vi "Modbus.vi"(8 "Command":string="\n", 10 "VISA资源名称":refnum<visa-resource-name>="COM1") -> (1 "响应":string)   [LabVIEW 2017]
uses:
  Program Files (x86)/National Instruments/LabVIEW 2017/examples/Instrument IO/Serial/support/Serial - Settings.ctl
  <vilib>/Instr/_visa.llb/VISA Configure Serial Port (Instr).vi
  <vilib>/NI/Modbus Library/API/Master/Modbus Master.lvclass
  <vilib>/NI/Modbus Library/API/Wrapper/Create Serial Master.vi
  <vilib>/NI/Modbus Library/API/Wrapper/API Main.lvlib
panel:
  out "字符串":string
  in  "register values 2":u16[](array[numeric])
  out "register values":u16[](array[numeric])
  out "error out":errorcluster
  in  "VISA resource name":refnum<visa-resource-name>
  out "Value 2":string
  out "Value":string
  out "子字符串":string
  in  "串口设置":T1={"波特率"=9600, "数据位"=8, "校验"=enum."None", "停止位"=10, "流控制"=0} {"流控制" items=["无"=0, "XON/XOFF"=1, "RTS/CTS"=2, "DTR/DSR"=4]; "停止位" items=["1.0"=10, "1.5"=15, "2.0"=20]; "数据位" min=5 max=8 step=1; "波特率" items=["75"=75, "110"=110, "134"=134, "150"=150, "300"=300, "600"=600, "1200"=1200, "1800"=1800, "2400"=2400, "4800"=4800, "7200"=7200, "9600"=9600, "14400"=14400, "19200"=19200, "28800"=28800, "38400"=38400, "56000"=56000, "57600"=57600, "115200"=115200, "128000"=128000, "230400"=230400]}
  in  "Command-Hex 2":string="*IDN?\n"
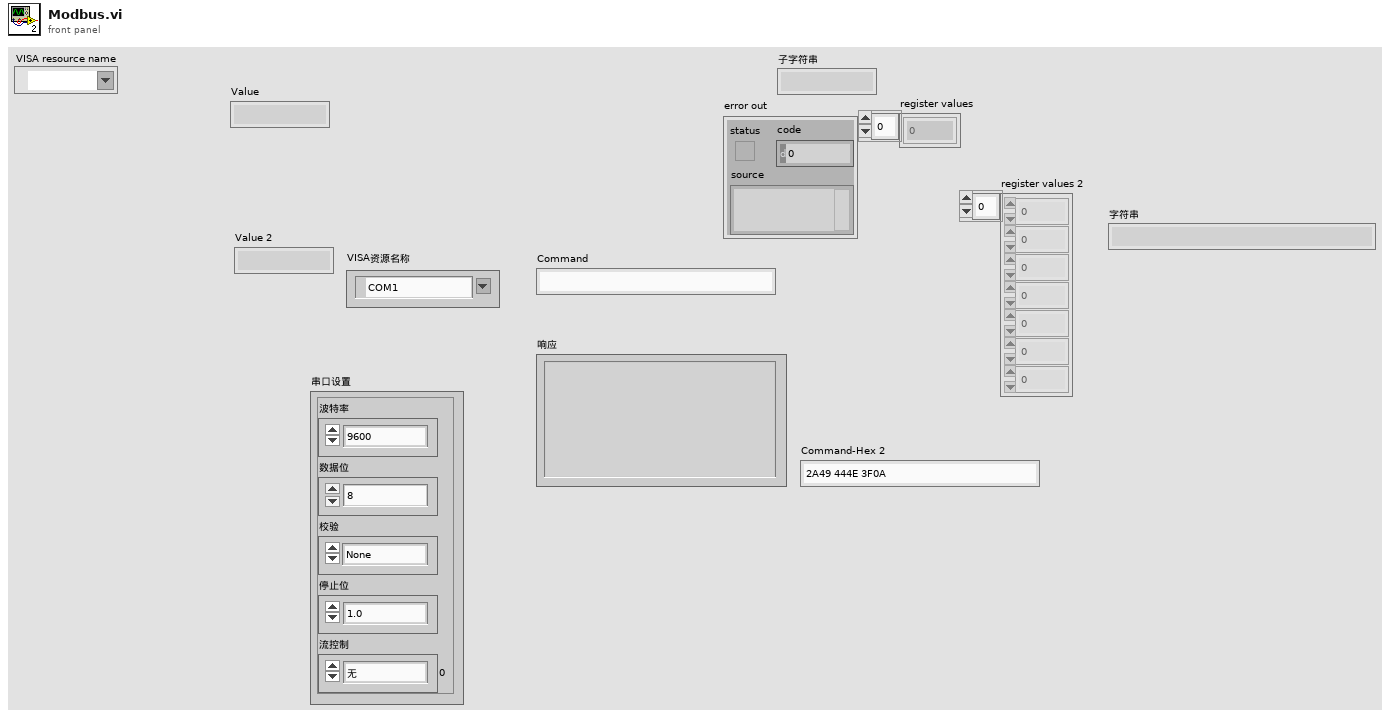
[diagram p1: front panel]
types:
  T1 = typedef "Serial - Settings.ctl" = cluster{"波特率":u32, "数据位":u16, "校验":enum16{"None", "Odd", "Even", "Mark", "Space"}, "停止位":u16, "流控制":u16}
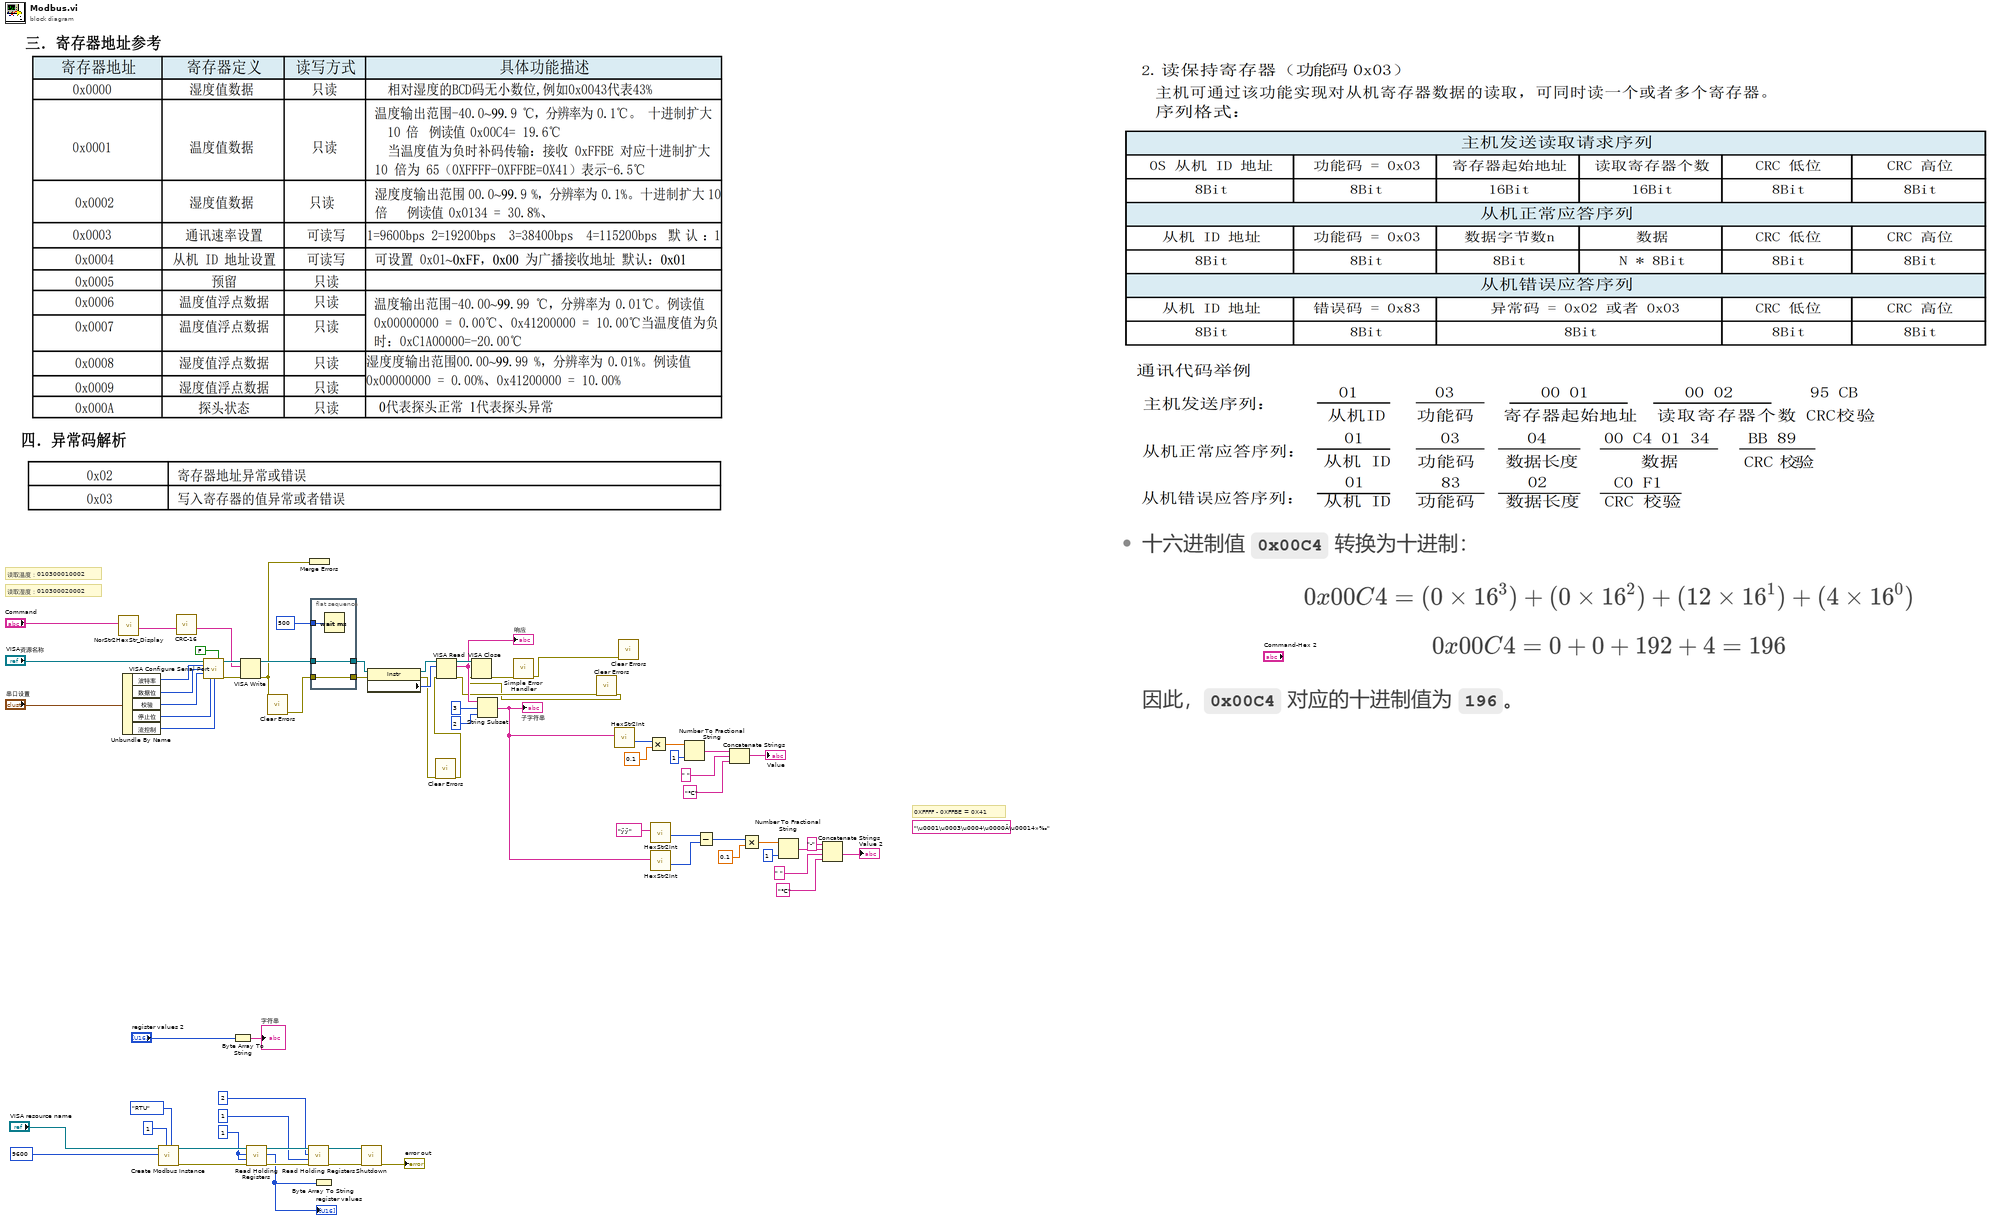
[diagram p0: block diagram]
diagram:
  w18 = u16 1 ("starting address")
  (unwired) "\u0001\u0003\u0004\u0000Ä\u00014»‰"
  # "0XFFFF - 0XFFBE = 0X41"
  # "读取湿度：010300020002"
  # "读取温度：010300010002"
  n1 = call "NorStr2HexStr_Display.vi"("Normal Display"="Command") -> ("Hex Display"=w50:string)  [unwired: 10 in]
  n2 = Unbundle By Name("串口设置") -> ("波特率"=w58:u32, "数据位"=w57:u16, "校验"=w56:enum16{"None", "Odd", "Even", "Mark", "Space"}, "停止位"=w55:u16, "流控制"=w54:u16)
  n3 = call-poly <vilib>:"Create Modbus Instance.vi"("serial type"=enum16{"RTU", "ASCII"}."RTU", "unit ID"=u8 1, "baud rate"=u32 9600, "VISA resource name"="VISA resource name") -> ("error out"=w19:errorcluster, "serial master instance"=w20:refnum<class "Modbus Master.lvclass">)  [unwired: 6 in]
  n4 = call "CRC-16.vi"("string_hex"=w50) -> ("string&CRC-16"=w7:string)  [unwired: 14 in]
  n5 = call-poly "VISA Configure Serial Port"("VISA resource name"="VISA资源名称", "Enable Termination\nChar (T)"=FALSE ("Enable Termination\nChar (T)"), "baud rate (9600)"=w58, "data bits (8)"=w57, "parity (0:none)"=w56, "stop bits (10: 1 bit)"=w55, "flow control (0:none)"=w54) -> ("VISA resource name out"=w67:refnum<visa-resource-name>, "error out"=w68:errorcluster)  [unwired: 2 in, 5 out]
  n6 = Byte Array To String(unsigned byte array="register values 2") -> (string=→"字符串":string)
  n7 = VISA Write(VISA resource name=w67, write buffer=w7, error in (no error)=w68) -> (VISA resource name out=w64:refnum<visa-resource-name>, error out=w3:errorcluster)  [unwired: 1 out]
  n8 = call-dynamic "Read Holding Registers.vi"("error in"=w19, "number of inputs"=w18, "starting address"=w18, "Modbus master in"=w20) -> ("error out"=w16:errorcluster, "register values"=w11:u16[], "Modbus master out"=w17:refnum<class "Modbus Master.lvclass">)  [unwired: 5 in]
  "register values" <- w11
  n9 = call <vilib>:"Clear Errors.vi"("error in (no error)"=w3) -> ("error out"=w6:errorcluster)  [unwired: 5 in, 1 out]
  n10 = call-dynamic "Read Holding Registers.vi"("error in"=w16, "number of inputs"=u16 1 ("starting address"), "starting address"=u16 2, "Modbus master in"=w17) -> ("error out"=w14:errorcluster, "Modbus master out"=w15:refnum<class "Modbus Master.lvclass">)  [unwired: 5 in, 1 out]
  n11 = Merge Errors(w3) -> ()  [unwired: 1 out]
  n12 = flat-sequence {
    tunnel: w6 -> [w71]
    tunnel: [w71] -> w65
    tunnel: w64 -> [w70]
    tunnel: [w70] -> w63
    tunnel: u32 500 ("读取前延时(ms)") -> [w72]
    frame #0 {
      n13 = Wait (ms)(milliseconds to wait=w72) -> ()  [unwired: 1 out]
    }
  }
  n14 = Byte Array To String(unsigned byte array=w11) -> ()  [unwired: 1 out]
  n15 = call-dynamic "Shutdown.vi"("error in"=w14, "Modbus master in"=w15) -> ("error out"=→"error out":errorcluster)  [unwired: 9 in]
  n16 = property class="Instr"(reference=w63, error in=w65) -> (reference out=w61:refnum<visa-resource-name>, error out=w10:errorcluster, "Serial Settings:Number of Bytes at Serial Port"=w60:u32)
  n17 = call <vilib>:"Clear Errors.vi"("error in (no error)"=w10) -> ("error out"=w5:errorcluster)  [unwired: 5 in, 1 out]
  n18 = VISA Read(VISA resource name=w61, byte count=w60, error in (no error)=w5) -> (VISA resource name out=w66:refnum<visa-resource-name>, read buffer=w47:string, error out=w9:errorcluster)  [unwired: 1 out]
  "响应" <- w47
  n19 = String Subset(string=w47, offset (0)=3 ("偏移量(0)"), length (rest)=2 ("长度（剩余）")) -> (substring=w26:string)
  "子字符串" <- w26
  n20 = call <vilib>:"Clear Errors.vi"("error in (no error)"=w9) -> ("error out"=w4:errorcluster)  [unwired: 5 in, 1 out]
  n21 = VISA Close(VISA resource name=w66, error in (no error)=w4) -> (error out=w52:errorcluster)
  n22 = call <vilib>:"Simple Error Handler.vi"("error in (no error)"=w52) -> ("error out"=w8:errorcluster)  [unwired: 1 in, 7 out]
  n23 = call "HexStr2Int.vi"("十六进制字符串"=w26) -> ("数字"=w46:u32)  [unwired: 10 in]
  n24 = call <vilib>:"Clear Errors.vi"("error in (no error)"=w8) -> ()  [unwired: 5 in, 2 out]
  n25 = Multiply(x=w46, y=0.1) -> (x*y=w44:dbl)
  n26 = call "HexStr2Int.vi"("十六进制字符串"="ÿÿ") -> ("数字"=w37:u32)  [unwired: 10 in]
  n27 = call "HexStr2Int.vi"("十六进制字符串"=w26) -> ("数字"=w36:u32)  [unwired: 10 in]
  n28 = Number To Fractional String(number=w44, precision (6)=i16 1 ("精度(6)")) -> (F-format string=w39:string)  [unwired: 2 in]
  n29 = Subtract(x=w37, y=w36) -> (x-y=w28:u32)
  n30 = Concatenate Strings(w39, " " ("字符串"), "℃" ("字符串")) -> (→"Value":string)
  n31 = Multiply(x=w28, y=0.1) -> (x*y=w30:dbl)
  n32 = Number To Fractional String(number=w30, precision (6)=i16 1 ("精度(6)")) -> (F-format string=w35:string)  [unwired: 2 in]
  n33 = Concatenate Strings("-" ("字符串"), w35, " " ("字符串"), "℃" ("字符串")) -> (→"Value 2":string)
